vi "Command.vi"(11 "Connection ID":T1) -> (3 "Connection ID Out":T1)   [LabVIEW 2017, in "GL860_Driver.lvlib"]
uses:
  GL860_Driver.lvlib
  Driver/ConnectionID.ctl
  Driver/GLdrv_RW.ctl
panel:
  in  "message 01":string="パネルを閉じますか？"
  in  "Clear":bool
  in  "Send":bool
  in  "Exit":bool
  in  "Text":string=">"
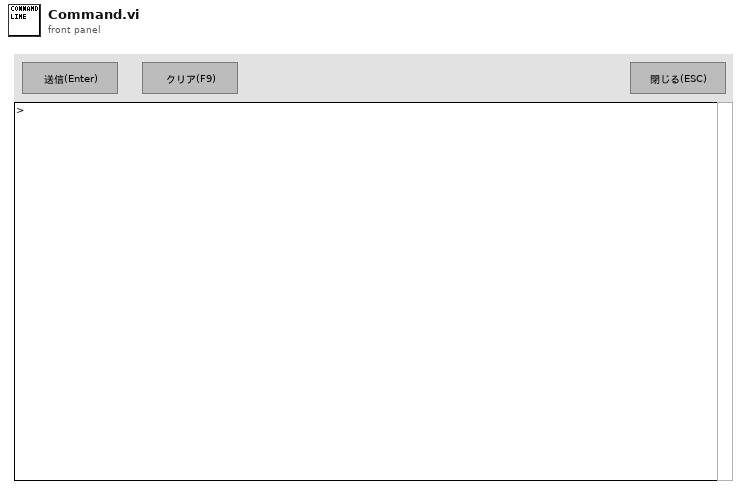
[diagram p1: front panel]
types:
  T1 = typedef "ConnectionID.ctl" = cluster{"Mode":enum16{"TCP/IP", "USB"}, "TCP/IP":refnum<k5>, "USB":i32}
  T2 = typedef "GLdrv_RW.ctl" = enum16{"Auto", "Read", "Write", "Buffer"}
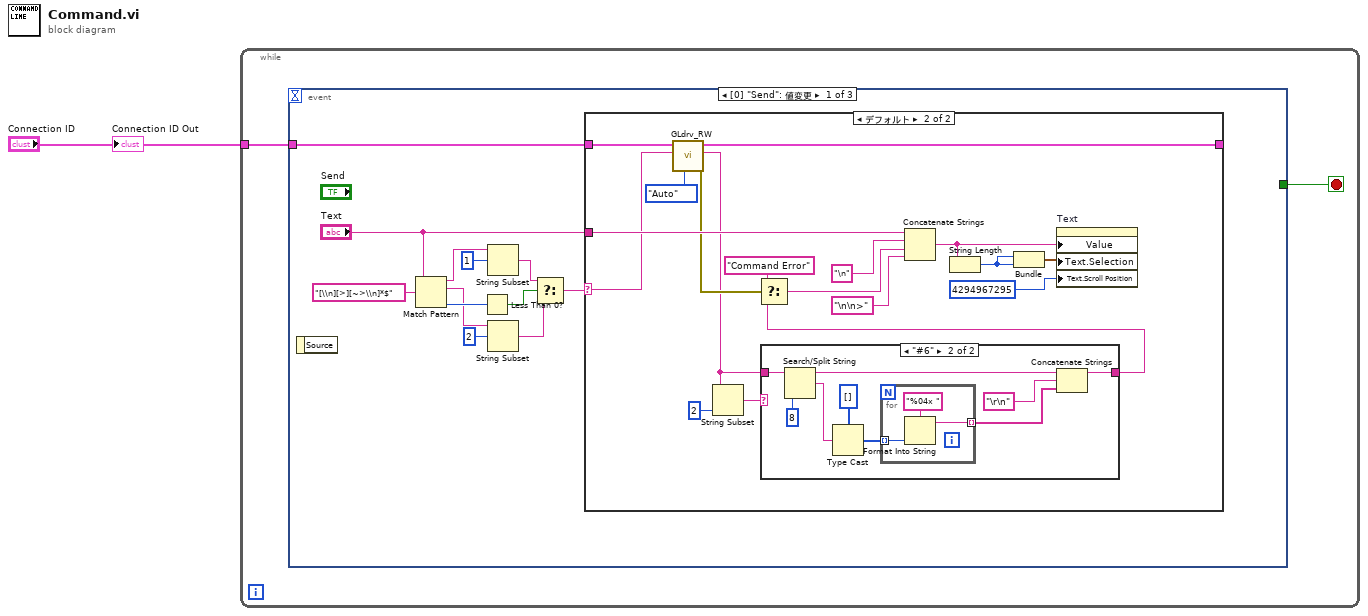
[diagram p0: block diagram]
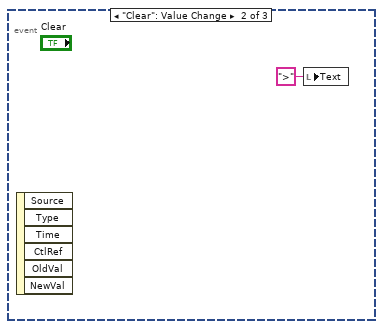
[diagram p4: hidden frame]
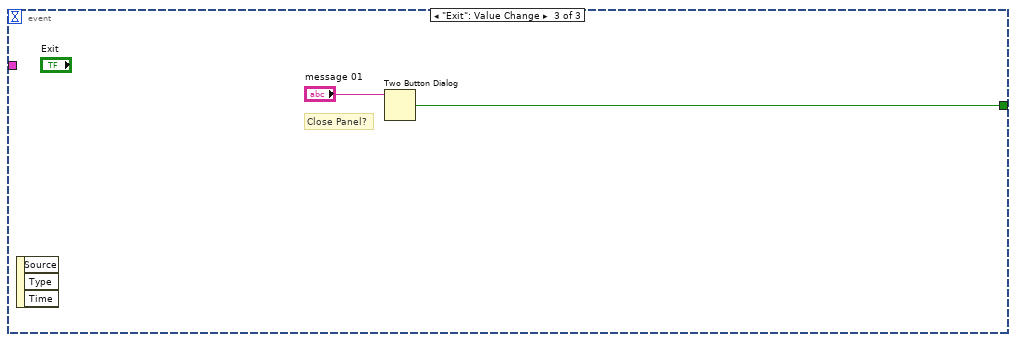
[diagram p5: hidden frame]
diagram:
  n1 = while {
    tunnel: "Connection ID" -> [w3]
    stop <- w2 stop-if-true
    n2 = event shown="[0] \"Send\": 値変更" {
      selector: _ -> [_ _ _]
      dyn-events: _ -> [_ _ _]
      timeout: _ -> [_ _ _]
      tunnel: w3 -> [w15 _ _]
      tunnel: [_ _ w49] -> w2
      event "Send": Value Change {
        n3 = event-data() -> ()  [unwired: 1 in, 1 out]
        n4 = Match Pattern(string="Text", regular expression="[\\n][>][~>\\n]*$") -> (before substring=w6:string, match substring=w10:string, offset past match=w12:i32)  [unwired: 1 in, 1 out]
        n5 = Less Than 0?(x=w12) -> (x < 0?=w11:bool)
        n6 = String Subset(string=w6, offset (0)=1) -> (substring=w5:string)  [unwired: 1 in]
        n7 = String Subset(string=w10, offset (0)=2) -> (substring=w8:string)  [unwired: 1 in]
        n8 = Select(t=w5, s=w11, f=w8) -> (s? t:f=w7:string)
        n9 = case shown="デフォルト" w7 {
          selector: w7 -> [_ w27]
          tunnel: w15 -> [w16 w34]
          tunnel: [w16 w33] -> _
          tunnel: "Text" -> [_ w32]
          frame "" {
          }
          frame Default {
            n10 = call "GLdrv_RW.vi"("Mode(read)"=GLdrv_RW."Auto", "data in"=w27, "Connection ID"=w34) -> ("error out"=w26:errorcluster, "data out"=w18:string, "Connection ID Out"=w33:T1)  [unwired: 4 in, 2 out]
            n11 = String Subset(string=w18, length (rest)=2 ("length (rest)")) -> (substring=w20:string)  [unwired: 1 in]
            n12 = case shown="\"#6\"" w20 {
              tunnel: w18 -> [w35 w41]
              tunnel: [w35 w42] -> w17
              frame Default {
              }
              frame "#6" {
                n13 = Search/Split String(string=w41, offset (0)=8) -> (substring before match=w37:string, match + rest of string=w40:string)  [unwired: 1 in, 1 out]
                n14 = Type Cast(type=u16[] [], x=w40) -> (*(type *) &x=w44:u16[])
                n15 = for {
                  tunnel: w44 -> [w47] mode=indexing
                  tunnel: [w46] -> w43 mode=indexing
                  n16 = Format Into String(format string="%04x ", w47) -> (resulting string=w46:string)  [unwired: 2 in, 1 out]
                }
                n17 = Concatenate Strings(w37, "\r\n" ("format string"), w43) -> (w42:string)
              }
            }
            n18 = Select(t="Command Error", s=w26, f=w17) -> (s? t:f=w25:string)
            n19 = Concatenate Strings(w32, "\n" ("string"), w25, "\n\n>" ("string")) -> (w28:string)
            n20 = String Length(string=w28) -> (length=w23:i32)
            n21 = Bundle(w23, w23) -> (w29:cluster{i32, i32})  [unwired: 1 in]
            n22 = property on="Text" class="Str"("Value"=w28, "Text.Selection"=w29, "Text.Scroll Position"=u32 4294967295) -> ()  [unwired: 2 in, 2 out]
          }
        }
      }
      event "Clear": Value Change {
        n23 = event-data() -> ()  [unwired: 1 in, 6 out]
        n24 = local write "Text"(">" ("Text")) -> ()
      }
      event "Exit": Value Change {
        # "Close Panel?"
        n25 = event-data() -> ()  [unwired: 1 in, 3 out]
        n26 = Two Button Dialog(message="message 01") -> (T button?=w49:bool)  [unwired: 2 in]
      }
    }
  }
  "Connection ID Out" <- "Connection ID"
